vi "booleanfunctions.vi"() -> ()   [LabVIEW 2015]
panel:
  in  "stop":bool
  out "coerced(x)":dbl
  out "In Range?":bool
  in  "upper limit":dbl
  in  "x":dbl
  in  "lower limit":dbl
  in  "Multicolumn Listbox":i32(listbox)
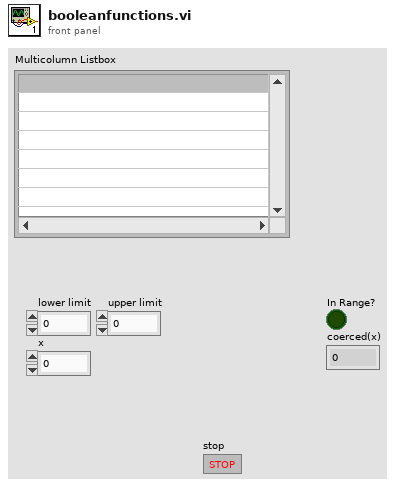
[diagram p1: front panel]
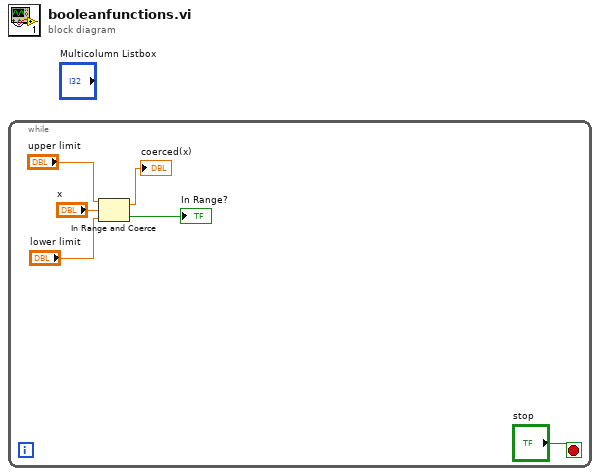
[diagram p0: block diagram]
diagram:
  n1 = while {
    stop <- "stop" stop-if-true
    n2 = In Range and Coerce(upper limit="upper limit", x="x", lower limit="lower limit") -> (coerced(x)=→"coerced(x)":dbl, In Range?=→"In Range?":bool)
  }
